vi "create_LS350_Data_header_units.vi"() -> (3 "String":string)   [LabVIEW 2018]
uses:
  Instrument_Setup.vi
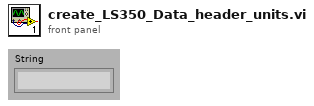
[diagram p1: front panel]
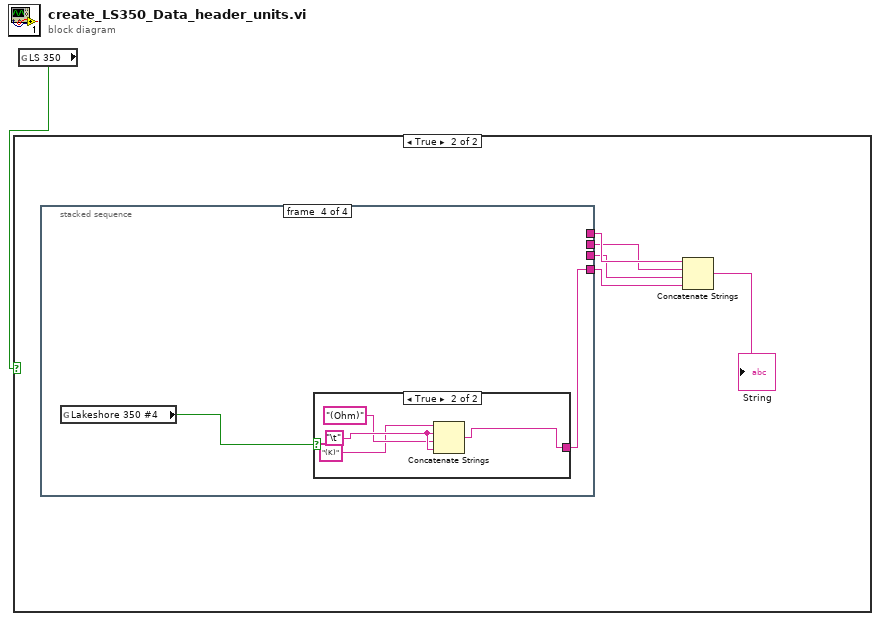
[diagram p0: block diagram]
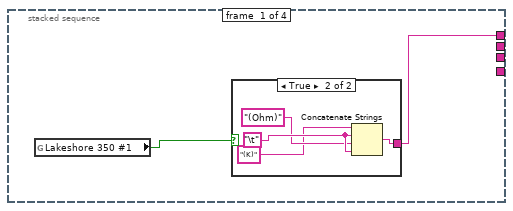
[diagram p3: hidden frame]
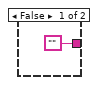
[diagram p4: hidden frame]
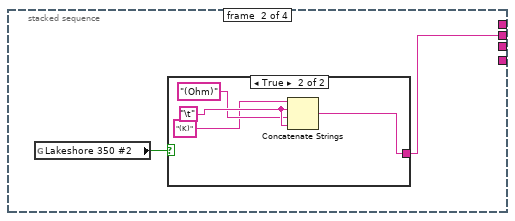
[diagram p5: hidden frame]
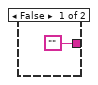
[diagram p6: hidden frame]
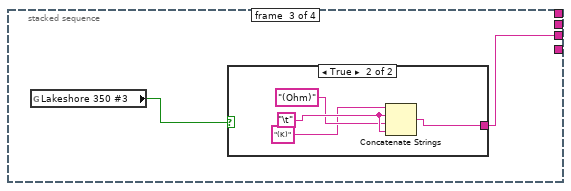
[diagram p7: hidden frame]
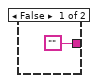
[diagram p8: hidden frame]
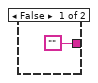
[diagram p9: hidden frame]
diagram:
  n1 = global read "Instrument_Setup.vi" "LS 350"() -> (w1:bool)
  n2 = case shown="True" w1 {
    frame False {
    }
    frame True {
      n3 = stacked-sequence {
        tunnel: [w7 _ _ _] -> w6
        tunnel: [_ w14 _ _] -> w5
        tunnel: [_ _ w21 _] -> w4
        tunnel: [_ _ _ w28] -> w3
        frame #0 {
          n4 = global read "Instrument_Setup.vi" "Lakeshore 350 #1"() -> (w8:bool)
          n5 = case shown="True" w8 {
            tunnel: ["" w13] -> w7
            frame False {
            }
            frame True {
              w12 = "\t"
              n6 = Concatenate Strings("(K)", w12, "(Ohm)", w12) -> (w13:string)
            }
          }
        }
        frame #1 {
          n7 = global read "Instrument_Setup.vi" "Lakeshore 350 #2"() -> (w15:bool)
          n8 = case shown="True" w15 {
            tunnel: ["" w19] -> w14
            frame False {
            }
            frame True {
              w20 = "\t"
              n9 = Concatenate Strings("(K)", w20, "(Ohm)", w20) -> (w19:string)
            }
          }
        }
        frame #2 {
          n10 = global read "Instrument_Setup.vi" "Lakeshore 350 #3"() -> (w22:bool)
          n11 = case shown="True" w22 {
            tunnel: ["" w26] -> w21
            frame False {
            }
            frame True {
              w27 = "\t"
              n12 = Concatenate Strings("(K)", w27, "(Ohm)", w27) -> (w26:string)
            }
          }
        }
        frame #3 {
          n13 = global read "Instrument_Setup.vi" "Lakeshore 350 #4"() -> (w29:bool)
          n14 = case shown="True" w29 {
            tunnel: ["" w33] -> w28
            frame False {
            }
            frame True {
              w34 = "\t"
              n15 = Concatenate Strings("(K)", w34, "(Ohm)", w34) -> (w33:string)
            }
          }
        }
      }
      n16 = Concatenate Strings(w6, w5, w4, w3) -> (→"String":string)
    }
  }
